vi "MAT Stream Writer Allign Streamed Data.vi"(5 "variable header offset (0: file start)":i64, 8 "error in (no error)":errorcluster, 9 "columns count":i32, 10 "rows count":i32, 11 "Ref Num":refnum<file>) -> (0 "error out":errorcluster, 1 "next var offset [B]":i64, 3 "Dup Ref Num":refnum<file>)   [LabVIEW 2020]
doc: "Matlab mat-v4 format lib: This VI should be used to fix header of the streamed variable after it is written. I.e. it will read the header of the streamed variable, updates rows and columns counts and writes it back. It also truncates file size so eventually preallocated data that are not used for the streamed variable are deleted. The variable is designated by its start offset in the file."
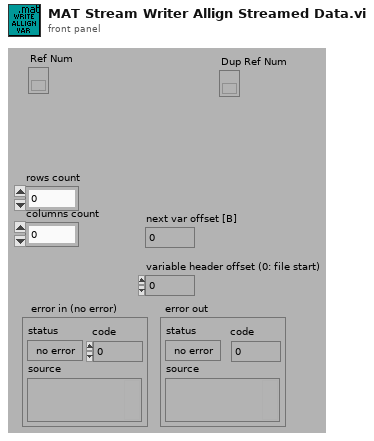
[diagram p1: front panel]
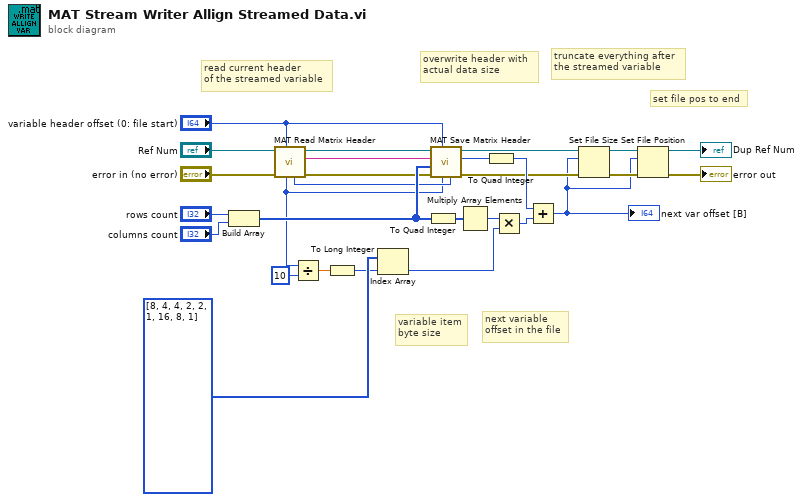
[diagram p0: block diagram]
diagram:
  # "set file pos to end"
  # "truncate everything after\nthe streamed variable"
  # "next variable\noffset in the file"
  # "overwrite header with\nactual data size"
  # "variable item\nbyte size"
  # "read current header\nof the streamed variable"
  n1 = Build Array("rows count", "columns count") -> (w25:i32[])
  n2 = call "MAT Read Matrix Header.vi"("offset in (-1: current position)"="variable header offset (0: file start)", "Error In"="error in (no error)", "Ref Num"="Ref Num") -> ("error out"=w20:errorcluster, "Matrix Name"=w16:string, "Dup Ref Num"=w18:refnum<file>, "Real/Complex (0 - Real)"=w15:u32, "Rep. Code"=w4:u32)  [unwired: 4 out]
  n3 = Divide(x=w4, y=u32 10) -> (x/y=w2:dbl)
  n4 = To Long Integer(number=w2) -> (32bit integer=w1:i32)
  n5 = Index Array(array=i32[] [8, 4, 4, 2, 2, 1, 16, 8, 1], index=w1) -> (element=w13:i32)
  n6 = To Quad Integer(1:w25) -> (0:w23:i64[])
  n7 = call "MAT Save Matrix Header.vi"("Real/Complex (0-Real)"=w15, "Rep. Code"=w4, "offset in (-1: current position)"="variable header offset (0: file start)", "error in (no error)"=w20, "Matrix Size"=w25, "Matrix Name"=w16, "Ref Num"=w18) -> ("error out"=w11:errorcluster, "offset out"=w24:i64, "Dup Ref Num"=w10:refnum<file>)  [unwired: 2 in]
  n8 = Multiply Array Elements(1:w23) -> (0:w14:i64)
  n9 = To Quad Integer(1:w24) -> (0:w22:i64)
  n10 = Multiply(x=w14, y=w13) -> (x*y=w12:i64)
  n11 = Add(x=w22, y=w12) -> (x+y=w5:i64)
  "next var offset [B]" <- w5
  n12 = Set File Size(4:w11, 6:w5, 7:w10) -> (0:w9:errorcluster, 3:w8:refnum<file>)
  n13 = Set File Position(offset (in bytes) (0)=w5, refnum=w8, error in=w9) -> (refnum out=→"Dup Ref Num":refnum<file>, error out=→"error out":errorcluster)  [unwired: 1 in]
